vi "applyInsertSpaceY.vi"(4 "deltaY":u16, 8 "error in (no error)":errorcluster, 10 "originY":i32, 11 "GObject in":refnum<class "GObject.lvclass">) -> (0 "error out":errorcluster, 3 "GObject out":refnum<class "GObject.lvclass">)   [LabVIEW 2023, in "TLC_Scripto.lvlib" / "GObject.lvclass"]
uses:
  GObject.lvclass
  GObject.lvclass/GObject.ctl
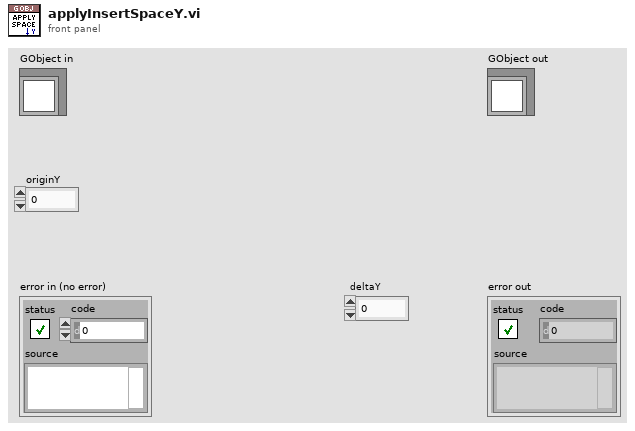
[diagram p1: front panel]
types:
  T1 = typedef "LVPositionTypeDef.ctl" = cluster{"Left":i32, "Top":i32}
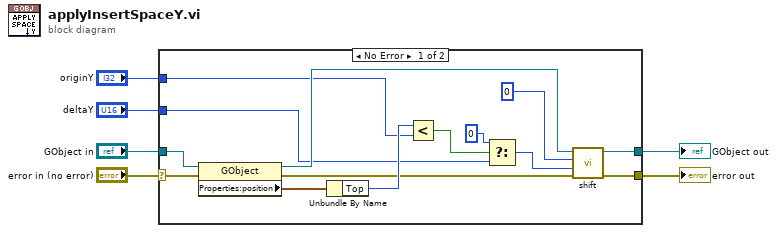
[diagram p0: block diagram]
diagram:
  n1 = case shown="No Error" "error in (no error)" {
    selector: "error in (no error)" -> [w8 w22]
    tunnel: [w15 w22] -> w5
    tunnel: [w13 w21] -> w3
    tunnel: "GObject in" -> [w12 w21]
    tunnel: "deltaY" -> [w14 _]
    tunnel: "originY" -> [w9 _]
    frame No Error {
      n2 = property class="GObject"(reference=w12, error in=w8) -> (reference out=w20:refnum<class "GObject.lvclass">, error out=w7:errorcluster, "Properties:position"=w19:T1)
      n3 = Unbundle By Name(w19) -> ("Top"=w18:i32)
      n4 = Less?(x=w18, y=w9) -> (x < y?=w17:bool)
      n5 = Select(t=u16 0, s=w17, f=w14) -> (s? t:f=w11:u16)
      n6 = call-dynamic "shift.vi"("error in (no error)"=w7, "deltaY[pixel]"=w11, "deltaX[pixel]"=0, "GObject in"=w20) -> ("error out"=w15:errorcluster, "GObject out"=w13:refnum<class "GObject.lvclass">)  [unwired: 6 in]
    }
    frame Error {
    }
  }
  "error out" <- w5
  "GObject out" <- w3
